vi "DBM_EndWork.vi"(8 "error in (no error)":errorcluster, 10 "Offset(min)":dbl, 11 "DBManager in":refnum<class "DBManager.lvclass">) -> (0 "error out":errorcluster, 3 "DBManager out":refnum<class "DBManager.lvclass">)   [LabVIEW 2015, in "DBManager.lvclass"]
uses:
  DBManager.lvclass
panel:
  # "Connector Pane"
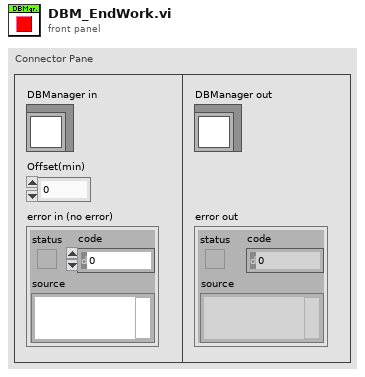
[diagram p1: front panel]
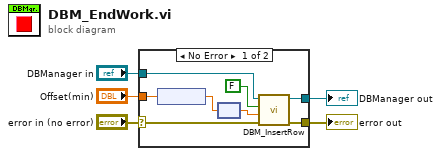
[diagram p0: block diagram]
diagram:
  n1 = case shown="No Error" "error in (no error)" {
    selector: "error in (no error)" -> [w11 w15]
    tunnel: [w10 w15] -> w4
    tunnel: [w12 w14] -> w2
    tunnel: "DBManager in" -> [w13 w14]
    tunnel: "Offset(min)" -> [w8 _]
    frame No Error {
      n2 = node(w8) -> (w7:dbl[unit])
      n3 = node(w7) -> (w6:dbl)
      n4 = call "DBM_InsertRow.vi"("error in (no error)"=w11, "Offset(s)"=w6, "IsStart?"=FALSE, "DBManager in"=w13) -> ("error out"=w10:errorcluster, "DBManager out"=w12:refnum<class "DBManager.lvclass">)  [unwired: 6 in]
    }
    frame Error {
    }
  }
  "error out" <- w4
  "DBManager out" <- w2
